vi "moveXY.vi"(1 "y position":i32, 2 "error in (no error)":errorcluster, 3 "x position":i32) -> (0 "error out":errorcluster)   [LabVIEW 2016]
uses:
  sa commands.ctl
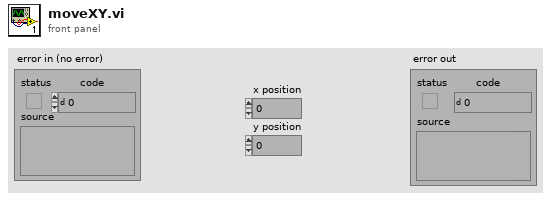
[diagram p1: front panel]
types:
  T1 = typedef "sa commands.ctl" = enum16{"read all", "set system index", "set x channel", "set y channel", "set rotation channel"}
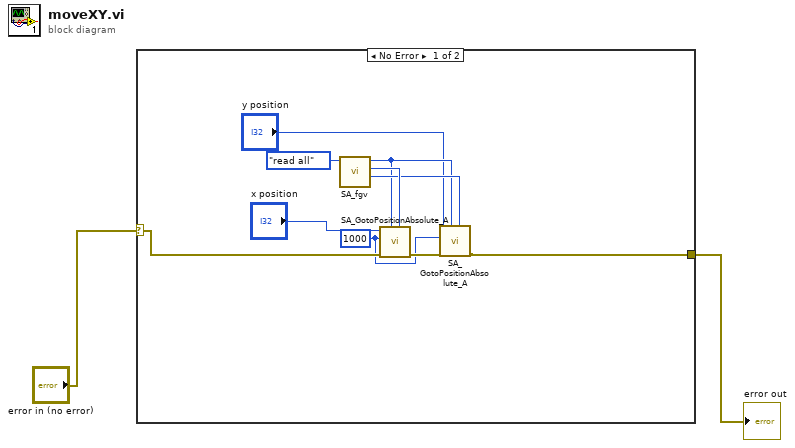
[diagram p0: block diagram]
diagram:
  n1 = case shown="No Error" "error in (no error)" {
    selector: "error in (no error)" -> [w12 w13]
    tunnel: [w9 w13] -> w1
    frame No Error {
      w4 = u32 1000 ("holdTime")
      n2 = call "SA_fgv.vi"("command"=sa_commands."read all") -> ("y channel"=w8:u32, "x channel"=w11:u32, "system index"=w7:u32)  [unwired: 3 in, 1 out]
      n3 = call <vilib>:"SA_GotoPositionAbsolute_A.vi"("channelIndex"=w11, "systemIndex"=w7, "error in (no error)"=w12, "holdTime"=w4, "position"="x position") -> ("error out"=w10:errorcluster)  [unwired: 6 in]
      n4 = call <vilib>:"SA_GotoPositionAbsolute_A.vi"("channelIndex"=w8, "systemIndex"=w7, "error in (no error)"=w10, "holdTime"=w4, "position"="y position") -> ("error out"=w9:errorcluster)  [unwired: 6 in]
    }
    frame Error {
    }
  }
  "error out" <- w1
